vi "TableIO.vi"(1 "IOSource":T2, 3 "Sample Time in":dbl format="%.10f", 4 "Table in":dbl[][](array[numeric]) format="%.4f", 5 "error in":errorcluster, 6 "Header in":T1={"Separator"="\t", "Remarks"="", "NDim"=0}, 7 "Names in":string[](array[string])) -> (12 "Header out":T1={"Separator"="\t", "Remarks"="", "NDim"=0}, 13 "Names out":string[](array[string]), 14 "Datastream out":string, 17 "Sample Time out":dbl format="%.10f", 18 "Table out":dbl[][](array[numeric]) format="%.2f", 19 "error out":errorcluster)   [LabVIEW 2020]
doc: "This VI reads or writes data files in table format. Sub-VI for DDL.vi, DRR?.vi, HIT?, GWD?.vi, JLT?.vi, TWS.vi etc. See separate manual GCSData User SM146E.pdf and control descriptions in the diagram for more information."
uses:
  Support.llb/GCSArray_regex_selector.ctl
  Support.llb/GCSArray_regex_range.ctl
panel:
  # "This vi reads or writes data files in table format. See separate manual \"GCSData User SM146E.pdf\" and control descriptions in the diagram for more information."
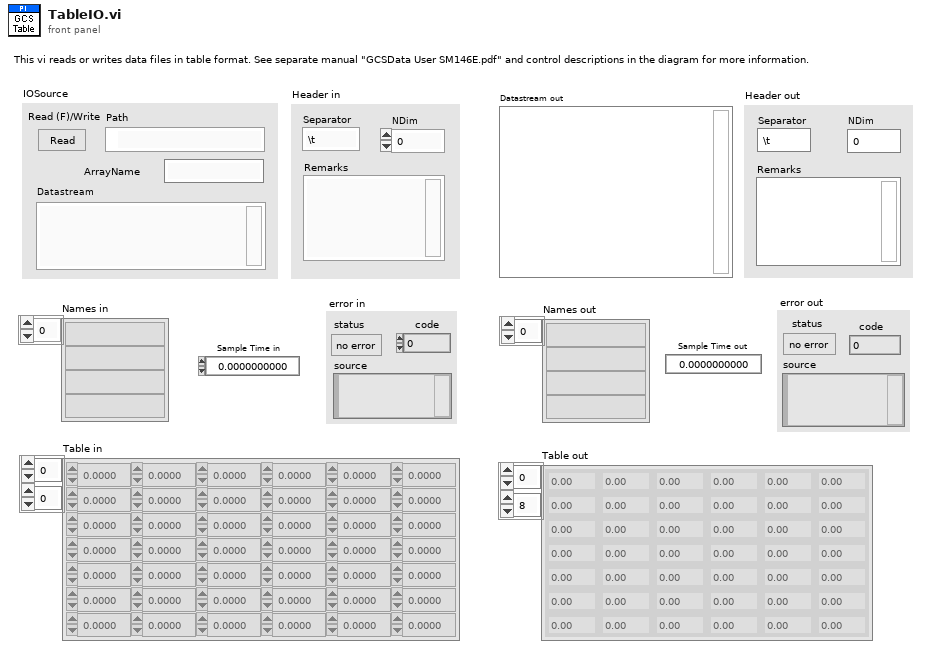
[diagram p1: front panel]
types:
  T1 = cluster{"Separator":string, "Remarks":string, "NDim":i32}
  T2 = cluster{"Read (F)/Write":bool, "Path":path, "Datastream":string, "ArrayName":string}
  T3 = enum16{"FirstTry", "Allocation", "FinalTry", "Native"}
  T4 = typedef "GCSArray_regex_range.ctl" = cluster{"Begin":i32, "End":i32}
  T5 = typedef "GCSArray_regex_selector.ctl" = enum16{"GCS_ARRAY Block Full", "GCS_ARRAY Block ID", "GCS_ARRAY Block Header", "GCS_ARRAY Block Data", "GCS_ARRAY Identifier", "GCS_ARRAY Remark", "GCS_ARRAY Version", "GCS_ARRAY Dimension", "GCS_ARRAY Type", "GCS_ARRAY Separator", "GCS_ARRAY NData", "GCS_ARRAY NData%", "GCS_ARRAY NData% Keyword", "GCS_ARRAY Name%", "GCS_ARRAY Name% Keyword", "GCS_ARRAY Start%", "GCS_ARRAY Start% Keyword", "GCS_ARRAY End%", "GCS_ARRAY End% Keyword", "GCS_ARRAY Delta%", "GCS_ARRAY Delta% Keword", "GCS_ARRAY Sample Time", "GCS_ARRAY Unit of transmitted value%", "GCS_ARRAY Trans_Unit% Keyword", "GCS_ARRAY Trans_Unit% = RAW Keyword", "GCS_ARRAY Unit of displayed value%", "GCS_ARRAY Disp_Unit% Keyword", "GCS_ARRAY Nominator%", "GCS_ARRAY Ratio_Nom% Keyword", "GCS_ARRAY Denominator%", "GCS_ARRAY Ratio_Denom% Keyword", "GCS_ARRAY End of Header", "GCS_ARRAY Empty line of Header"}
  T6 = typedef "GCSArray_header.ctl" = cluster{"Identifier":string, "Version":i32, "Remark":string, "Dimension":i32, "Type":enum16{"Matrix", "Table"}, "Separator":u8, "NData":i32, "NData%":i32[], "Name%":string[], "Start%":dbl[], "End%":dbl[], "Delta%":dbl[], "SampleTime":dbl, "TransmittedUnit%":string[], "DisplayedUnit%":string[], "RatioNominator%":dbl[], "RatioDenominator%":dbl[]}
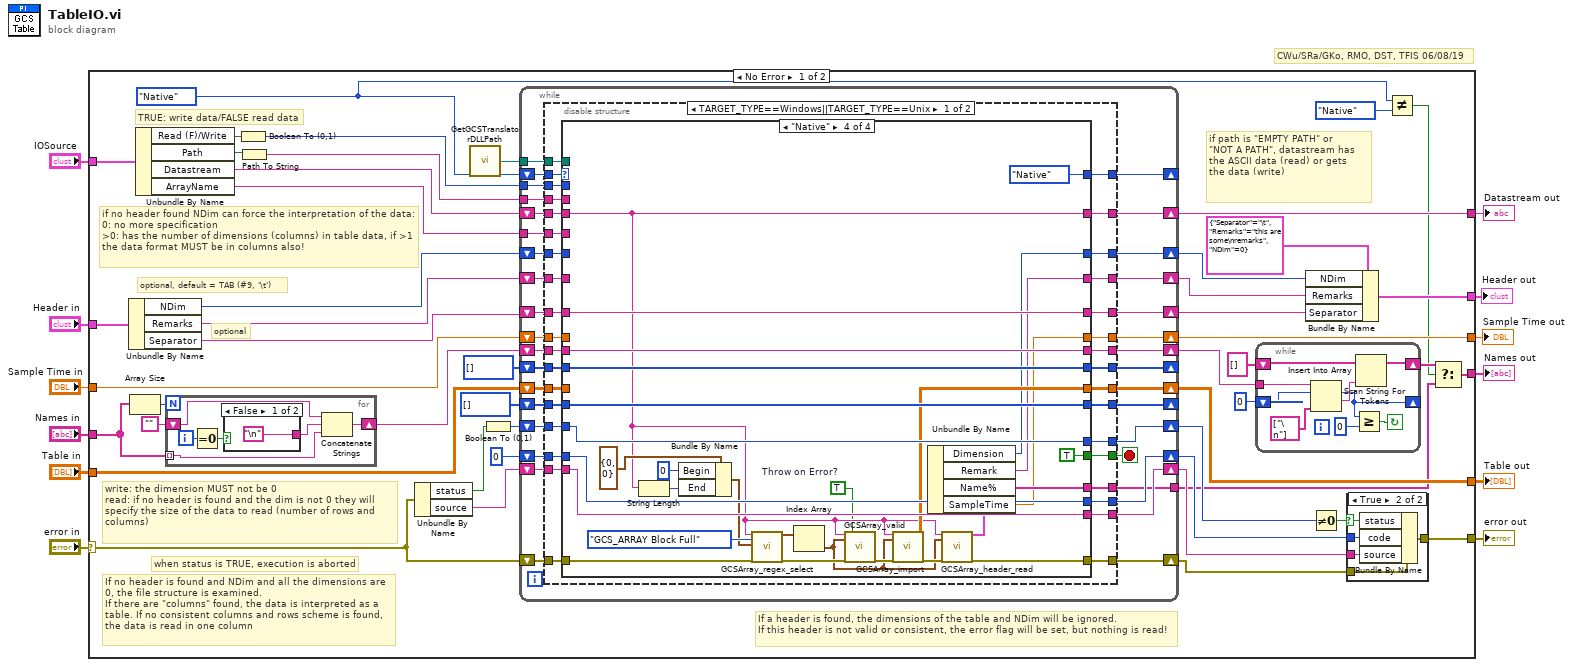
[diagram p0: block diagram]
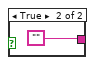
[diagram p2: hidden frame]
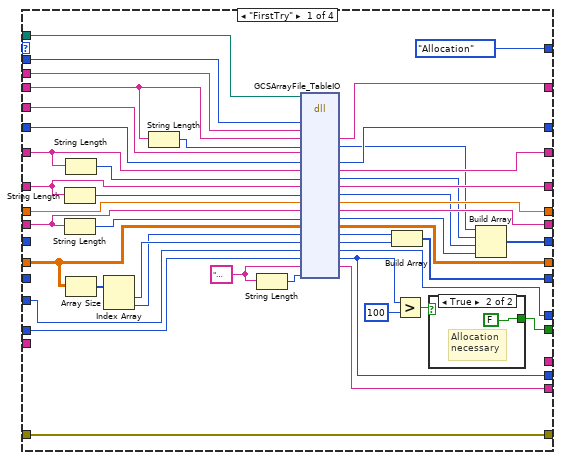
[diagram p3: hidden frame]
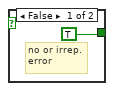
[diagram p4: hidden frame]
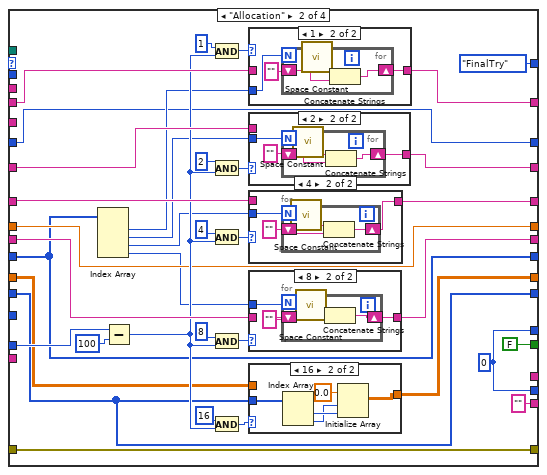
[diagram p5: hidden frame]
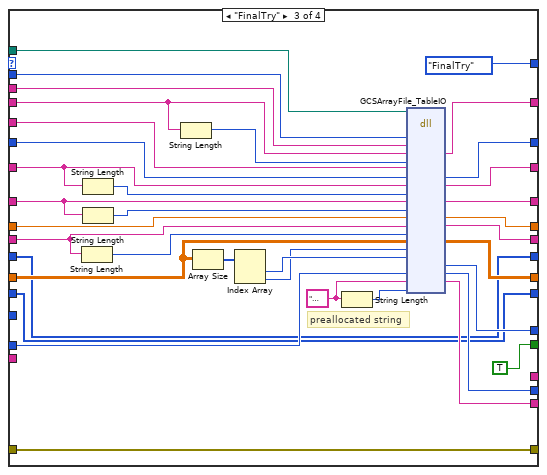
[diagram p11: hidden frame]
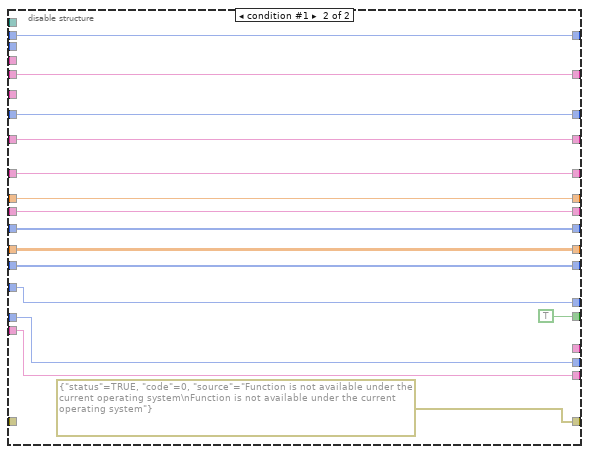
[diagram p12: hidden frame]
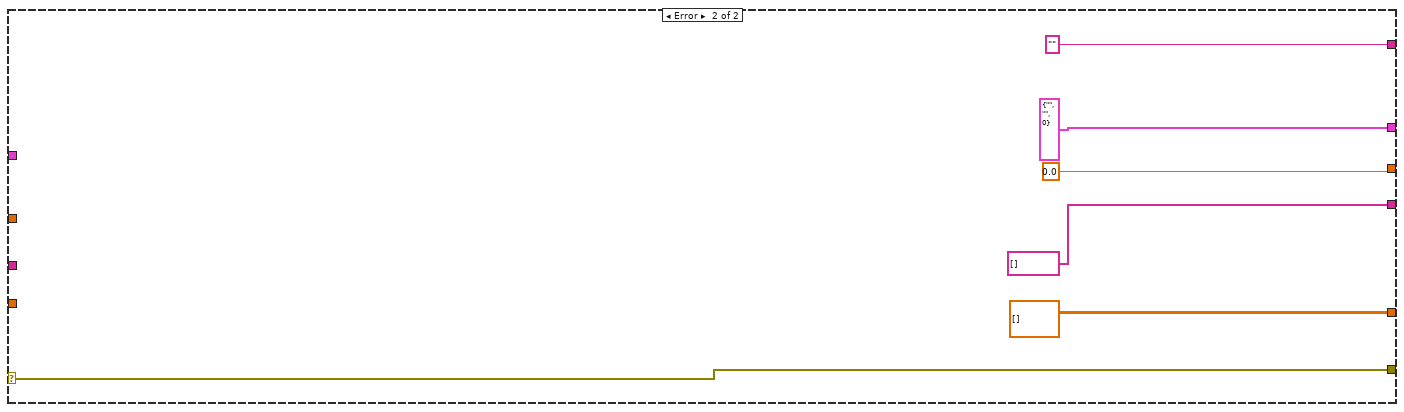
[diagram p14: hidden frame]
diagram:
  # "CWu/SRa/GKo, RMO, DST, TFIS 06/08/19"
  n1 = case shown="No Error" "error in" {
    selector: "error in" -> [w20 w349]
    tunnel: "IOSource" -> [w60 _]
    tunnel: "Header in" -> [w59 _]
    tunnel: [w57 T1 {"Separator"="", "Remarks"="", "NDim"=0} ("Header Out 2")] -> w10
    tunnel: "Table in" -> [w56 _]
    tunnel: "Sample Time in" -> [w49 _]
    tunnel: [w45 dbl[][] [] ("Table")] -> w7
    tunnel: [w43 w349] -> w6
    tunnel: [w40 "" ("DataStream")] -> w5
    tunnel: [w39 0.0 ("SampleTime")] -> w4
    tunnel: [w17 string[] []] -> w3
    tunnel: "Names in" -> [w34 _]
    frame No Error {
      w15 = T3."Native"
      # "If no header is found and NDim and all the dimensions are 0, the file structure is examined.\nIf there are \"columns\" found, the data is interpreted as a table. If no consistent columns and rows scheme is found, the data is read in one column"
      # "If a header is found, the dimensions of the table and NDim will be ignored.\nIf this header is not valid or consistent, the error flag will be set, but nothing is read!"
      # "write: the dimension MUST not be 0\nread: if no header is found and the dim is not 0 they will\nspecify the size of the data to read (number of rows and columns)"
      # "when status is TRUE, execution is aborted"
      # "optional, default = TAB (#9, '\\t')"
      # "optional"
      # "if no header found NDim can force the interpretation of the data:\n0: no more specification\n>0: has the number of dimensions (columns) in table data, if >1 the data format MUST be in columns also!"
      # "if path is \"EMPTY PATH\" or \n\"NOT A PATH\", datastream has \nthe ASCII data (read) or gets \nthe data (write)"
      # "TRUE: write data/FALSE read data"
      n2 = Unbundle By Name(w59) -> ("NDim"=w24:i32, "Remarks"=w50:string, "Separator"=w25:string)
      n3 = Array Size(array=w34) -> (size(s)=w32:i32)
      n4 = Unbundle By Name(w60) -> ("Read (F)/Write"=w55:bool, "Path"=w46:path, "Datastream"=w51:string, "ArrayName"=w52:string)
      n5 = for {
        N: w32 -> [_]
        shift-right: [w65] -> w31
        shift-left: "" -> [w66]
        tunnel: w34 -> [w63] mode=indexing
        i -> [w62]
        n6 = Equal To 0?(x=w62) -> (x = 0?=w61:bool)
        n7 = case shown="False" w61 {
          tunnel: ["\n" ""] -> w64
          frame False {
          }
          frame True {
          }
        }
        n8 = Concatenate Strings(w66, w64, w63) -> (w65:string)
      }
      n9 = Boolean To (0,1)(Boolean=w55) -> (0, 1=w54:i16)
      n10 = Path To String(path=w46) -> (string=w53:string)
      n11 = Unbundle By Name(w20) -> ("status"=w48:bool, "source"=w27:string)
      n12 = call "GetGCSTranslatorDLLPath.vi"() -> ("DLL path"=w21:path)  [unwired: 1 in]
      n13 = Boolean To (0,1)(Boolean=w48) -> (0, 1=w47:i16)
      n14 = while {
        tunnel: w54 -> [w110]
        tunnel: w53 -> [w109]
        tunnel: w52 -> [w108]
        shift-right: [w101] -> w22
        shift-left: w24 -> [w106]
        shift-right: [w100] -> w30
        shift-left: w50 -> [w105]
        shift-right: [w99] -> w23
        shift-left: w25 -> [w104]
        shift-right: [w98] -> w45
        shift-left: w56 -> [w111]
        shift-right: [w96] -> w38
        shift-left: w47 -> [w102]
        shift-right: [w97] -> w44
        shift-left: 0 ("errorcode") -> [w94]
        shift-right: [w92] -> _
        shift-left: w15 -> [w93]
        shift-right: [w90] -> w40
        shift-left: w51 -> [w107]
        shift-right: [w89] -> w35
        shift-left: w31 -> [w86]
        shift-right: [w88] -> _
        shift-left: u32[] [] -> [w87]
        shift-right: [w84] -> _
        shift-left: u32[] [] -> [w83]
        shift-right: [w95] -> w41
        shift-left: w27 -> [w82]
        shift-right: [w85] -> w39
        shift-left: w49 -> [w103]
        tunnel: w21 -> [w81]
        shift-right: [w80] -> w19
        shift-left: w20 -> [w79]
        tunnel: [w78] -> w16
        stop <- w91 stop-if-true
        n15 = disable-structure shown="TARGET_TYPE==Windows||TARGET_TYPE==Unix" {
          disable-tunnel: w111 -> [w145 w334]
          disable-tunnel: w110 -> [w144 _]
          disable-tunnel: w109 -> [w143 _]
          disable-tunnel: w108 -> [w142 _]
          disable-tunnel: w107 -> [w141 w342]
          disable-tunnel: w106 -> [w140 w340]
          disable-tunnel: w105 -> [w139 w339]
          disable-tunnel: w104 -> [w138 w338]
          disable-tunnel: w103 -> [w137 w337]
          disable-tunnel: w102 -> [w136 w332]
          disable-tunnel: [w135 w340] -> w101
          disable-tunnel: [w134 w339] -> w100
          disable-tunnel: [w133 w338] -> w99
          disable-tunnel: [w132 w334] -> w98
          disable-tunnel: [w131 w331] -> w97
          disable-tunnel: [w130 w332] -> w96
          disable-tunnel: [w129 w330] -> w95
          disable-tunnel: w94 -> [w128 w331]
          disable-tunnel: w93 -> [w127 w341]
          disable-tunnel: [w126 w341] -> w92
          disable-tunnel: [w125 TRUE] -> w91
          disable-tunnel: [w124 w342] -> w90
          disable-tunnel: [w123 w336] -> w89
          disable-tunnel: [w122 w335] -> w88
          disable-tunnel: w87 -> [w121 w335]
          disable-tunnel: w86 -> [w120 w336]
          disable-tunnel: [w119 w337] -> w85
          disable-tunnel: [w118 w333] -> w84
          disable-tunnel: w83 -> [w117 w333]
          disable-tunnel: w82 -> [w116 w330]
          disable-tunnel: w81 -> [w115 _]
          disable-tunnel: [w114 errorcluster {"status"=TRUE, "code"=0, "source"="Function is not available under the current operating system\nFunction is not available under the current operating system"} ("error IO")] -> w80
          disable-tunnel: w79 -> [w113 _]
          disable-tunnel: [w112 _] -> w78
          frame condition #0 (active) {
            n16 = case shown="\"Native\"" w127 {
              tunnel: w145 -> [w158 w205 w298 _]
              tunnel: w144 -> [w190 _ w297 _]
              tunnel: w143 -> [w189 _ w296 _]
              tunnel: w142 -> [w188 _ w295 _]
              tunnel: w141 -> [w187 w222 w294 w301]
              tunnel: w140 -> [w186 w197 w293 _]
              tunnel: w139 -> [w185 w219 w271 _]
              tunnel: w138 -> [w184 w215 w292 w326]
              tunnel: w137 -> [w183 w202 w291 _]
              tunnel: w136 -> [w182 _ _ w322]
              tunnel: [w181 w197 w290 w308] -> w135
              tunnel: [w180 w218 w289 w307] -> w134
              tunnel: [w179 w214 w288 w326] -> w133
              tunnel: [w156 w206 w287 w311] -> w132
              tunnel: [w159 w195 w286 w320] -> w131
              tunnel: [w154 w195 w285 w322] -> w130
              tunnel: [w178 "" ("errorsource") w284 w319] -> w129
              tunnel: w128 -> [w177 w227 w283 w320]
              tunnel: [T3."Allocation" T3."FinalTry" T3."FinalTry" T3."Native"] -> w126
              tunnel: [w152 FALSE TRUE TRUE] -> w125
              tunnel: [w157 w223 w274 w301] -> w124
              tunnel: [w171 w211 w277 w325] -> w123
              tunnel: [w165 w194 w265 w324] -> w122
              tunnel: w121 -> [_ w194 w265 w324]
              tunnel: w120 -> [w168 w210 w275 w325]
              tunnel: [w169 w202 w276 w305] -> w119
              tunnel: [w155 w196 w266 w323] -> w118
              tunnel: w117 -> [_ w196 w266 w323]
              tunnel: w116 -> [_ _ _ w319]
              tunnel: w115 -> [w147 _ w264 _]
              tunnel: [w146 w193 w263 w304] -> w114
              tunnel: w113 -> [w146 w193 w263 w318]
              tunnel: [_ _ _ w306] -> w112
              frame "FirstTry" {
                w173 = "                                                                                                                                             " ("string")
                n17 = String Length(string=w184) -> (length=w149:i32)
                n18 = String Length(string=w168) -> (length=w148:i32)
                n19 = String Length(string=w185) -> (length=w150:i32)
                n20 = Array Size(array=w158) -> (size(s)=w176:i32[])
                n21 = Index Array(array=w176) -> (element #1=w175:i32, element #2=w174:i32)  [unwired: 2 in]
                n22 = String Length(string=w187) -> (length=w151:i32)
                n23 = String Length(string=w173) -> (length=w172:i32)
                n24 = dll-call lib="T:/Entwicklung/HostSoftware/LabVIEW/GCSDrivers/source/GCS2LabVIEW/Low Level/GCSTranslator.dll" fn="GCSArrayFile_TableIO"(path in=w147, "WriteAccess"=w190, "Path"=w189, "DataStream"=w187, "DataStreamBufferSize"=w151, "ArrayName"=w188, "NDim"=w186, "Remarks"=w185, "RemarksBufferSize"=w150, "Separator"=w184, "SeparatorBufferSize"=w149, "SampleTime"=w183, "Names"=w168, "NamesBufferSize"=w148, "Table"=w158, "TableColumns"=w174, "TableRows"=w175, "errorstatus"=w182, "errorcode"=w177, "errorsource"=w173, "errorsrcbufsize"=w172) -> ("DataStream"=w157:string, "DataStreamBufferSize"=w162:u32, "NDim"=w181:u32, "Remarks"=w180:string, "RemarksBufferSize"=w163:u32, "Separator"=w179:string, "SeparatorBufferSize"=w164:u32, "SampleTime"=w169:dbl, "Names"=w171:string, "NamesBufferSize"=w170:u32, "Table"=w156:dbl[][], "TableColumns"=w167:u32, "TableRows"=w166:u32, "errorstatus"=w154:u8, "errorcode"=w159:i32, "errorsource"=w178:string)  [unwired: 5 in, 4 out]
                n25 = Build Array(w167, w166) -> (w155:u32[])
                n26 = Greater?(x=w159, y=100 ("x")) -> (0:w161:bool)
                n27 = case shown="True" w161 {
                  tunnel: [TRUE FALSE] -> w152
                  frame False {
                    # "no or irrep.\nerror"
                  }
                  frame True {
                    # "Allocation\nnecessary"
                  }
                }
                n28 = Build Array(w162, w163, w164, w170) -> (w165:u32[])
              }
              frame "Allocation" {
                w195 = 0 ("errorcode")
                n29 = Index Array(array=w194) -> (element #1=w198:u32, element #2=w199:u32, element #3=w200:u32, element #4=w201:u32)  [unwired: 4 in]
                n30 = Subtract(x=w227, y=100) -> (x-y=w208:i32)
                n31 = And(x=1, y=w208) -> (x .and. y?=w224:i32)
                n32 = And(x=2, y=w208) -> (x .and. y?=w221:i32)
                n33 = And(x=4, y=w208) -> (x .and. y?=w217:i32)
                n34 = And(x=8, y=w208) -> (x .and. y?=w213:i32)
                n35 = And(x=16, y=w208) -> (x .and. y?=w209:i32)
                n36 = case shown="1" w224 {
                  tunnel: [w256 w258] -> w223
                  tunnel: w222 -> [w256 _]
                  tunnel: w198 -> [_ w257]
                  frame 0, Default {
                  }
                  frame 1 {
                    n37 = for {
                      N: w257 -> [_]
                      shift-right: [w261] -> w258
                      shift-left: "" -> [w260]
                      n38 = call <vilib>:"Space Constant.vi"() -> ("String"=w262:string)
                      n39 = Concatenate Strings(w262, w260) -> (w261:string)
                    }
                  }
                }
                n40 = case shown="2" w221 {
                  tunnel: [w249 w251] -> w218
                  tunnel: w219 -> [w249 _]
                  tunnel: w199 -> [_ w250]
                  frame 0, Default {
                  }
                  frame 2 {
                    n41 = for {
                      N: w250 -> [_]
                      shift-right: [w254] -> w251
                      shift-left: "" -> [w253]
                      n42 = call <vilib>:"Space Constant.vi"() -> ("String"=w255:string)
                      n43 = Concatenate Strings(w255, w253) -> (w254:string)
                    }
                  }
                }
                n44 = case shown="4" w217 {
                  tunnel: [w242 w244] -> w214
                  tunnel: w215 -> [w242 _]
                  tunnel: w200 -> [_ w243]
                  frame 0, Default {
                  }
                  frame 4 {
                    n45 = for {
                      N: w243 -> [_]
                      shift-right: [w247] -> w244
                      shift-left: "" -> [w246]
                      n46 = call <vilib>:"Space Constant.vi"() -> ("String"=w248:string)
                      n47 = Concatenate Strings(w248, w246) -> (w247:string)
                    }
                  }
                }
                n48 = case shown="8" w213 {
                  tunnel: [w235 w237] -> w211
                  tunnel: w210 -> [w235 _]
                  tunnel: w201 -> [_ w236]
                  frame 0, Default {
                  }
                  frame 8 {
                    n49 = for {
                      N: w236 -> [_]
                      shift-right: [w240] -> w237
                      shift-left: "" -> [w239]
                      n50 = call <vilib>:"Space Constant.vi"() -> ("String"=w241:string)
                      n51 = Concatenate Strings(w241, w239) -> (w240:string)
                    }
                  }
                }
                n52 = case shown="16" w209 {
                  tunnel: [w229 w234] -> w206
                  tunnel: w205 -> [w229 _]
                  tunnel: w196 -> [_ w232]
                  frame 0, Default {
                  }
                  frame 16 {
                    n53 = Index Array(array=w232) -> (element #1=w231:u32, element #2=w230:u32)  [unwired: 2 in]
                    n54 = Initialize Array(0.0 ("element"), w230, w231) -> (w234:dbl[][])
                  }
                }
              }
              frame "FinalTry" {
                w272 = "                                                                                                                                             " ("string")
                # "preallocated string"
                n55 = String Length(string=w275) -> (length=w268:i32)
                n56 = String Length(string=w271) -> (length=w270:i32)
                n57 = String Length(string=w292) -> (length=w269:i32)
                n58 = String Length(string=w294) -> (length=w267:i32)
                n59 = Array Size(array=w298) -> (size(s)=w282:i32[])
                n60 = Index Array(array=w282) -> (element #1=w281:i32, element #2=w280:i32)  [unwired: 2 in]
                n61 = String Length(string=w272) -> (length=w279:i32)
                n62 = dll-call lib="T:/Entwicklung/HostSoftware/LabVIEW/GCSDrivers/source/GCS2LabVIEW/Low Level/GCSTranslator.dll" fn="GCSArrayFile_TableIO"(path in=w264, "WriteAccess"=w297, "Path"=w296, "DataStream"=w294, "DataStreamBufferSize"=w267, "ArrayName"=w295, "NDim"=w293, "Remarks"=w271, "RemarksBufferSize"=w270, "Separator"=w292, "SeparatorBufferSize"=w269, "SampleTime"=w291, "Names"=w275, "NamesBufferSize"=w268, "Table"=w298, "TableColumns"=w280, "TableRows"=w281, "errorcode"=w283, "errorsource"=w272, "errorsrcbufsize"=w279) -> ("DataStream"=w274:string, "NDim"=w290:u32, "Remarks"=w289:string, "Separator"=w288:string, "SampleTime"=w276:dbl, "Names"=w277:string, "Table"=w287:dbl[][], "errorstatus"=w285:u8, "errorcode"=w286:i32, "errorsource"=w284:string)  [unwired: 9 in, 7 out]
              }
              frame "Native" {
                w299 = TRUE  # Throw on Error?
                n63 = String Length(string=w301) -> (length=w314:i32)
                n64 = Bundle By Name(cluster=T4 {"Begin"=0, "End"=0} ("Range"), "Begin"=0, "End"=w314) -> (w313:T4)
                n65 = call "GCSArray_regex_select.vi"("GCSArray input string"=w301, "Selector"=GCSArray_regex_selector."GCS_ARRAY Block Full", "Range"=w313, "error in (no error)"=w318) -> ("Matches"=w312:T4[], "error out"=w302:errorcluster)  [unwired: 14 out]
                n66 = Index Array(array=w312) -> (element=w300:T4)  [unwired: 1 in]
                n67 = call "GCSArray_valid.vi"("GCSArray input string"=w301, "Selection"=w300, "error in (no error)"=w302, "Throw on Error?"=w299) -> ("error out"=w303:errorcluster)  [unwired: 15 out]
                n68 = call "GCSArray_import.vi"("GCSArray input string"=w301, "Range"=w300, "error in (no error)"=w303) -> ("GCSArray data"=w311:dbl[][], "error out"=w310:errorcluster)  [unwired: 15 out]
                n69 = call "GCSArray_header_read.vi"("GCSArray input string"=w301, "Range"=w300, "error in (no error)"=w310) -> ("GCSArray Header"=w309:T6, "error out"=w304:errorcluster)  [unwired: 15 out]
                n70 = Unbundle By Name(w309) -> ("Dimension"=w308:i32, "Remark"=w307:string, "Name%"=w306:string[], "SampleTime"=w305:dbl)
              }
            }
          }
          frame condition #1 {
          }
        }
      }
      n71 = while {
        shift-right: [w75] -> w18
        shift-left: string[] [] -> [w74]
        shift-right: [w71] -> _
        shift-left: 0 ("offset past token") -> [w72]
        tunnel: w35 -> [w70]
        stop <- w76 continue-if-true
        n72 = Scan String For Tokens(6:string[] ["\n"] ("delimiters (\\s,\\t,\\r,\\n)"), 8:w72, 9:w70) -> (1:w73:string, 2:w71:i32)  [unwired: 5 out]
        n73 = Greater Or Equal?(x=w71, y=0) -> (x >= y?=w76:bool)
        n74 = Insert Into Array(array=w74, new element=w73) -> (w75:string[])  [unwired: 1 in]
      }
      n75 = Bundle By Name(cluster=T1 {"Separator"="\t", "Remarks"="this are some\nremarks", "NDim"=0} ("Header Out 2"), "NDim"=w22, "Remarks"=w30, "Separator"=w23) -> (w57:T1)
      n76 = Not Equal To 0?(x=w38) -> (x != 0?=w42:bool)
      n77 = case shown="True" w42 {
        selector: w42 -> [_ w344]
        tunnel: w44 -> [_ w348]
        tunnel: w41 -> [_ w346]
        tunnel: [w343 w347] -> w43
        tunnel: w19 -> [w343 w345]
        frame False {
        }
        frame True {
          n78 = Bundle By Name(cluster=w345, "status"=w344, "code"=w348, "source"=w346) -> (w347:errorcluster)
        }
      }
      n79 = Not Equal?(x=w15, y=T3."Native") -> (x != y?=w13:bool)
      n80 = Select(t=w18, s=w13, f=w16) -> (s? t:f=w17:string[])
    }
    frame Error {
    }
  }
  "error out" <- w6
  "Datastream out" <- w5
  "Header out" <- w10
  "Names out" <- w3
  "Table out" <- w7
  "Sample Time out" <- w4
